vi "CLD 12 Sequencer State Machine.vi"() -> ()   [LabVIEW 2019]
doc: "CLD 12 exercise"
uses:
  CLD 12 Data Cluster.ctl
  CLD 12 Sequencer Enum.ctl
  CLD12 Timer Enum.ctl
panel:
  in  "Start":bool
  out "Data Out 2":T1[](array[typedef])
  out "Current Time Target":dbl
  in  "Stop Button":bool
  out "Time Elapsed":dbl
  out "Switch 3":bool
  out "Switch 2":bool
  out "Switch 1":bool
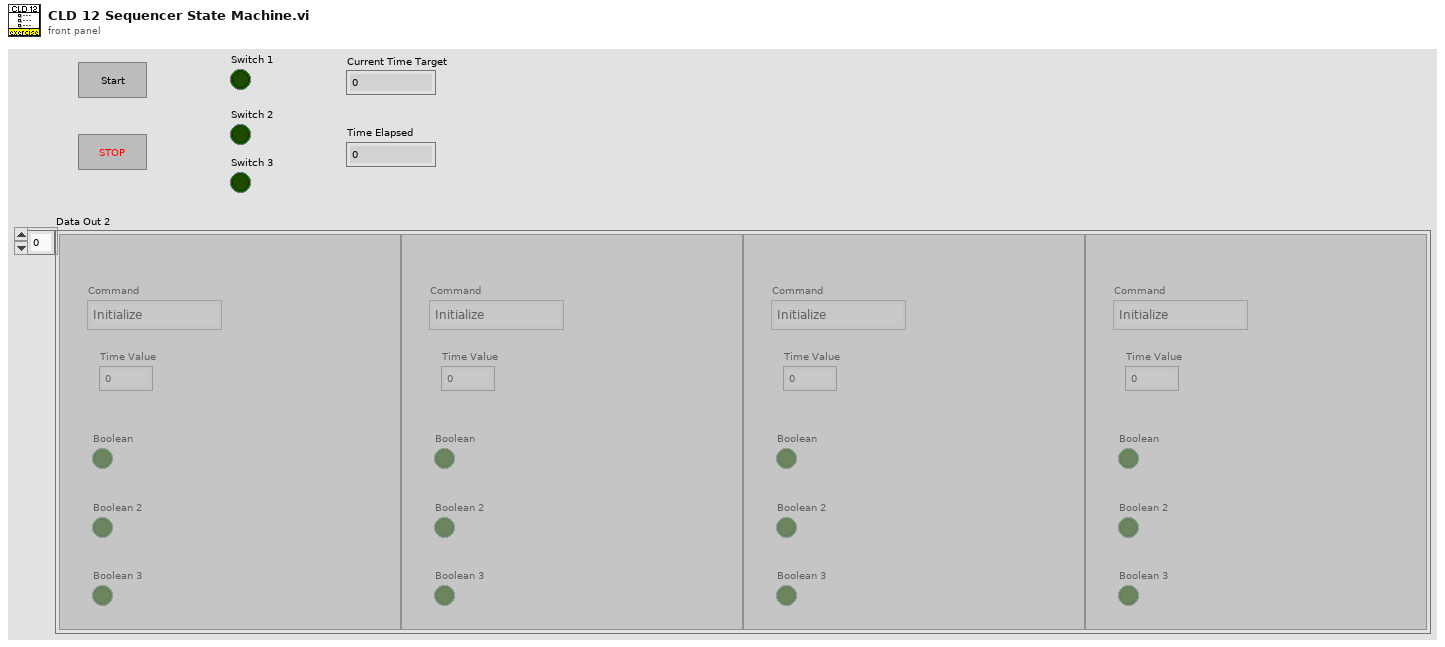
[diagram p1: front panel]
types:
  T1 = typedef "CLD 12 Data Cluster.ctl" = cluster{"Command":T2, "Time Value":dbl, "Boolean":bool, "Boolean 2":bool, "Boolean 3":bool}
  T2 = typedef "CLD 12 Sequencer Enum.ctl" = enum16{"Initialize", "SetTime", "RunState1", "Runstate2", "Idle", "Start"}
  T3 = typedef "CLD12 Timer Enum.ctl" = enum16{"Start Timer", "Reset Timer", "Read Time", "Pause", "Resume"}
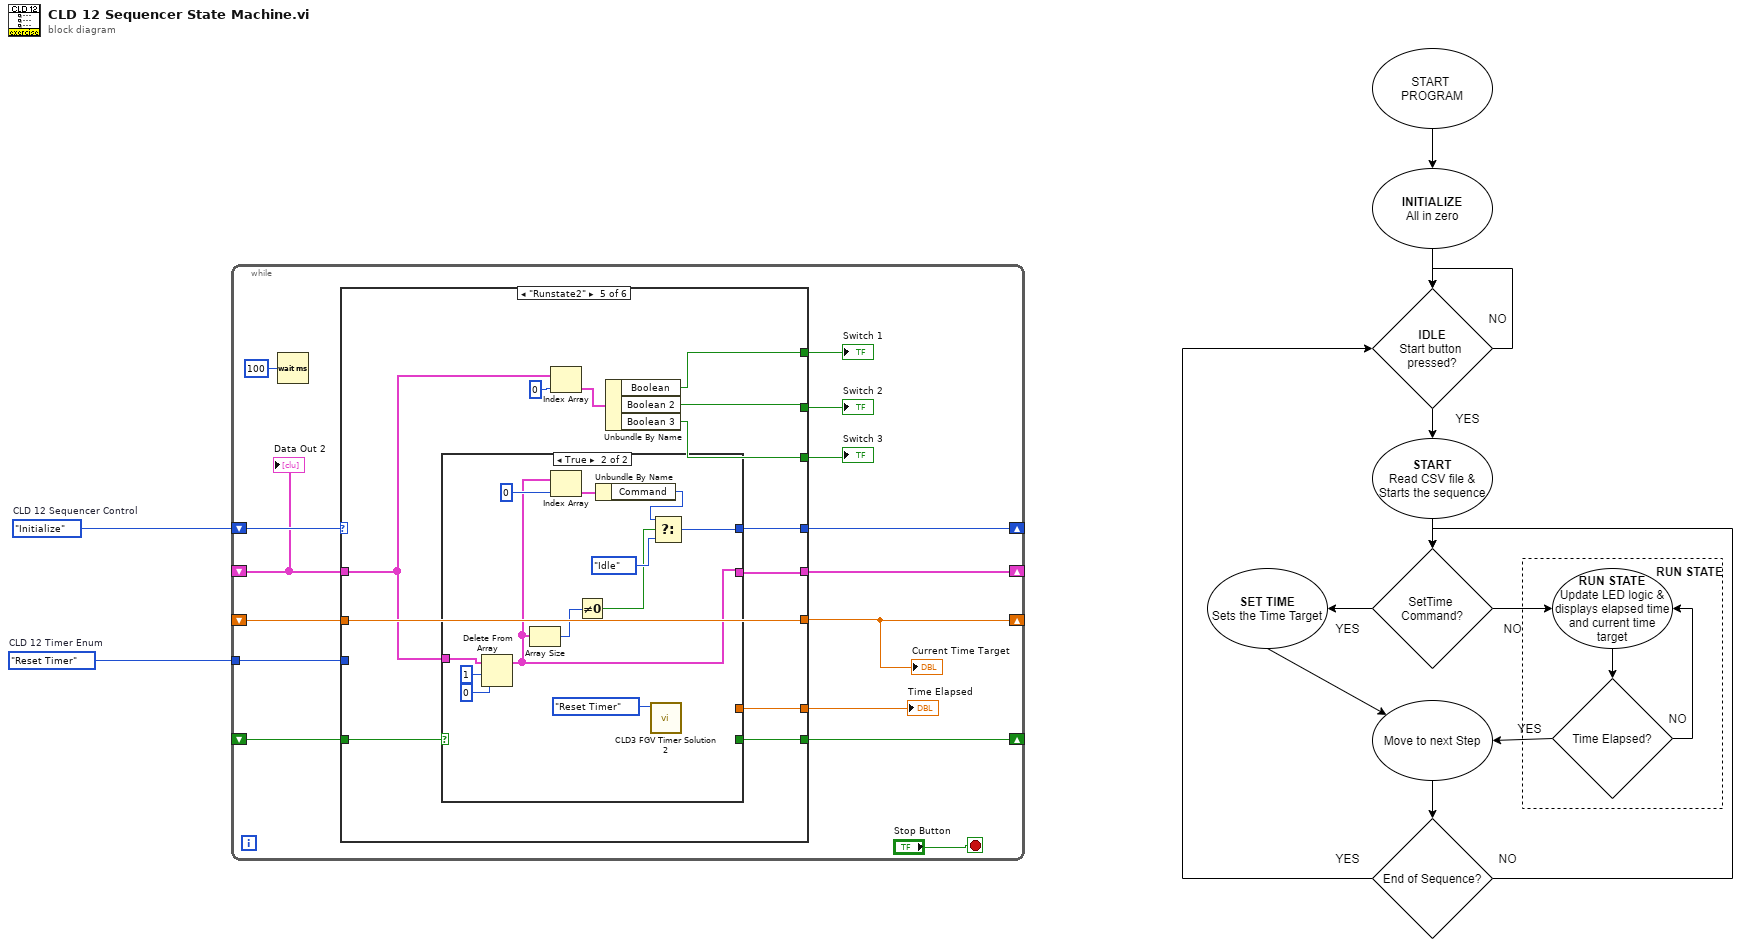
[diagram p0: block diagram]
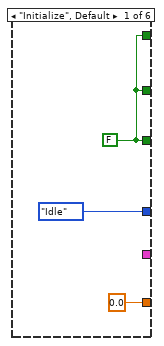
[diagram p2: hidden frame]
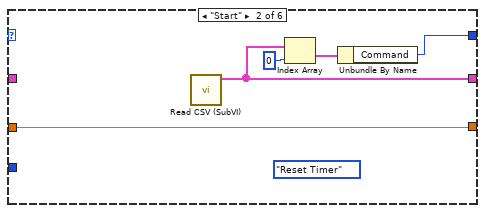
[diagram p3: hidden frame]
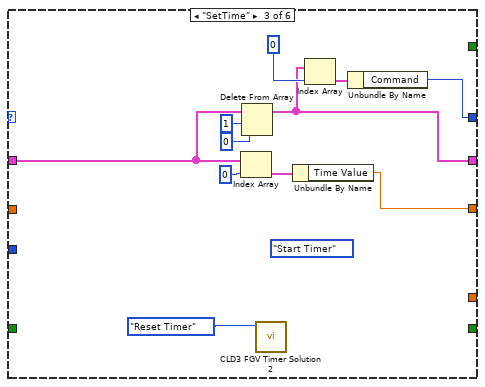
[diagram p4: hidden frame]
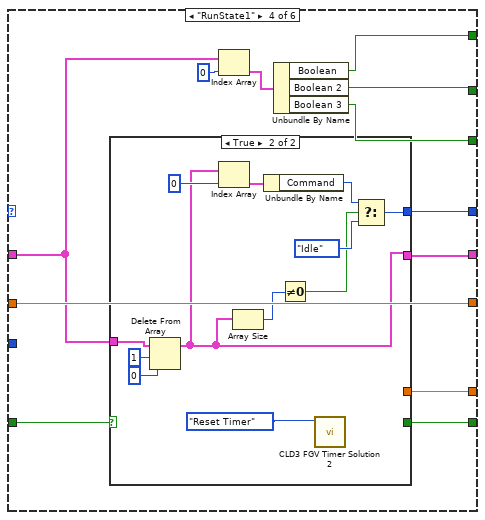
[diagram p5: hidden frame]
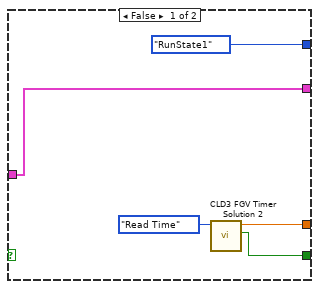
[diagram p6: hidden frame]
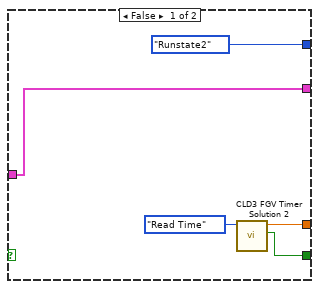
[diagram p7: hidden frame]
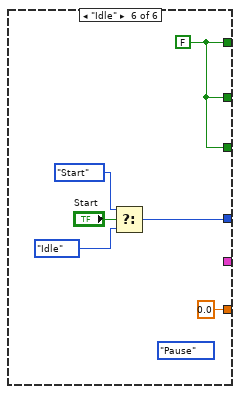
[diagram p8: hidden frame]
diagram:
  w2 = CLD_12_Sequencer_Enum."Initialize"  # CLD 12 Sequencer Control
  w1 = CLD12_Timer_Enum."Reset Timer"  # CLD 12 Timer Enum
  n1 = while {
    shift-right: [w16] -> _
    shift-left: w2 -> [w17]
    tunnel: w1 -> [w11]
    shift-right: [w12] -> _
    shift-left: _ -> [w8]
    shift-right: [w9] -> _
    shift-left: _ -> [w10]
    shift-right: [w5] -> _
    shift-left: _ -> [w4]
    stop <- "Stop Button" stop-if-true
    n2 = Wait (ms)(milliseconds to wait=u32 100) -> ()  [unwired: 1 out]
    n3 = case shown="\"Runstate2\"" w17 {
      tunnel: [CLD_12_Sequencer_Enum."Idle" ("CLD 12 Sequencer Control") w22 w28 w40 w69 w95] -> w16
      tunnel: [w20 _ _ w45 w74 w100] -> w15
      tunnel: [w20 _ _ w44 w73 w100] -> w14
      tunnel: [w20 _ _ w43 w72 w100] -> w13
      tunnel: [_ w24 w27 w41 w70 _] -> w12
      tunnel: w11 -> [_ _ _ _ _ _]
      tunnel: [0.0 ("Current Time Target") w21 w35 w48 w77 0.0 ("Current Time Target")] -> w9
      tunnel: w10 -> [_ w21 _ w48 w77 _]
      tunnel: w8 -> [_ _ w34 w42 w71 _]
      tunnel: [_ _ _ w39 w68 _] -> w6
      tunnel: [_ _ _ w37 w67 _] -> w5
      tunnel: w4 -> [_ _ _ w38 w66 _]
      frame "Initialize", Default {
        w20 = FALSE ("Switch 3")
      }
      frame "Start" {
        (unwired) CLD12_Timer_Enum."Reset Timer" ("CLD 12 Timer Enum")
        n4 = call "Read CSV (SubVI).vi"() -> ("Data Out"=w24:T1[])  [unwired: 11 in]
        n5 = Index Array(array=w24, index=0) -> (element=w23:T1)
        n6 = Unbundle By Name(w23) -> ("Command"=w22:T2)
      }
      frame "SetTime" {
        (unwired) CLD12_Timer_Enum."Start Timer" ("CLD 12 Timer Enum")
        n7 = Index Array(array=w34, index=0) -> (element=w31:T1)
        n8 = Delete From Array(array=w34, length=1, index=0) -> (array with subset deleted=w27:T1[])  [unwired: 1 out]
        n9 = call "CLD3 FGV Timer Solution 2.vi"("Timer Mode"=CLD12_Timer_Enum."Reset Timer" ("CLD 12 Timer Enum")) -> ()  [unwired: 8 in, 3 out]
        n10 = Unbundle By Name(w31) -> ("Time Value"=w35:dbl)
        n11 = Index Array(array=w27, index=0) -> (element=w29:T1)
        n12 = Unbundle By Name(w29) -> ("Command"=w28:T2)
      }
      frame "RunState1" {
        n13 = case shown="True" w38 {
          tunnel: w42 -> [w53 w61]
          tunnel: [w53 w60] -> w41
          tunnel: [CLD_12_Sequencer_Enum."RunState1" ("CLD 12 Sequencer Control") w58] -> w40
          tunnel: [w50 _] -> w39
          tunnel: [w49 _] -> w37
          frame False {
            n14 = call "CLD3 FGV Timer Solution 2.vi"("Timer Mode"=CLD12_Timer_Enum."Read Time" ("CLD 12 Timer Enum")) -> ("Has Time Elapsed"=w49:bool, "Elapsed Time (s.ss)"=w50:dbl)  [unwired: 8 in, 1 out]
          }
          frame True {
            n15 = Delete From Array(array=w61, length=1, index=0) -> (array with subset deleted=w60:T1[])  [unwired: 1 out]
            n16 = Index Array(array=w60, index=0) -> (element=w62:T1)
            n17 = Array Size(array=w60) -> (size(s)=w59:i32)
            n18 = Unbundle By Name(w62) -> ("Command"=w57:T2)
            n19 = Not Equal To 0?(x=w59) -> (x != 0?=w55:bool)
            n20 = call "CLD3 FGV Timer Solution 2.vi"("Timer Mode"=CLD12_Timer_Enum."Reset Timer" ("CLD 12 Timer Enum")) -> ()  [unwired: 8 in, 3 out]
            n21 = Select(t=w57, s=w55, f=CLD_12_Sequencer_Enum."Idle" ("CLD 12 Sequencer Control")) -> (s? t:f=w58:T2)
          }
        }
        n22 = Index Array(array=w42, index=0) -> (element=w46:T1)
        n23 = Unbundle By Name(w46) -> ("Boolean"=w45:bool, "Boolean 2"=w44:bool, "Boolean 3"=w43:bool)
      }
      frame "Runstate2" {
        n24 = case shown="True" w66 {
          tunnel: w71 -> [w82 w90]
          tunnel: [w82 w84] -> w70
          tunnel: [CLD_12_Sequencer_Enum."Runstate2" ("CLD 12 Sequencer Control") w86] -> w69
          tunnel: [w79 _] -> w68
          tunnel: [w78 _] -> w67
          frame False {
            n25 = call "CLD3 FGV Timer Solution 2.vi"("Timer Mode"=CLD12_Timer_Enum."Read Time" ("CLD 12 Timer Enum")) -> ("Has Time Elapsed"=w78:bool, "Elapsed Time (s.ss)"=w79:dbl)  [unwired: 8 in, 1 out]
          }
          frame True {
            n26 = Delete From Array(array=w90, length=1, index=0) -> (array with subset deleted=w84:T1[])  [unwired: 1 out]
            n27 = Array Size(array=w84) -> (size(s)=w89:i32)
            n28 = Index Array(array=w84, index=0) -> (element=w91:T1)
            n29 = Not Equal To 0?(x=w89) -> (x != 0?=w87:bool)
            n30 = Unbundle By Name(w91) -> ("Command"=w85:T2)
            n31 = call "CLD3 FGV Timer Solution 2.vi"("Timer Mode"=CLD12_Timer_Enum."Reset Timer" ("CLD 12 Timer Enum")) -> ()  [unwired: 8 in, 3 out]
            n32 = Select(t=w85, s=w87, f=CLD_12_Sequencer_Enum."Idle" ("CLD 12 Sequencer Control")) -> (s? t:f=w86:T2)
          }
        }
        n33 = Index Array(array=w71, index=0) -> (element=w75:T1)
        n34 = Unbundle By Name(w75) -> ("Boolean"=w74:bool, "Boolean 2"=w73:bool, "Boolean 3"=w72:bool)
      }
      frame "Idle" {
        (unwired) CLD12_Timer_Enum."Pause" ("CLD 12 Timer Enum")
        w100 = FALSE ("Boolean")
        n35 = Select(t=CLD_12_Sequencer_Enum."Start" ("CLD 12 Sequencer Control"), s="Start", f=CLD_12_Sequencer_Enum."Idle" ("CLD 12 Sequencer Control")) -> (s? t:f=w95:T2)
      }
    }
    "Time Elapsed" <- w6
    "Current Time Target" <- w9
    "Switch 1" <- w15
    "Switch 2" <- w14
    "Switch 3" <- w13
    "Data Out 2" <- w8
  }
